vi "sub_filter_n_offset.vi"(8 "error in":errorcluster, 10 "offset?":bool, 11 "Q_data":T2) -> (0 "error out":errorcluster, 2 "data out":T1)   [LabVIEW 2013]
uses:
  ctl/q_data.ctl
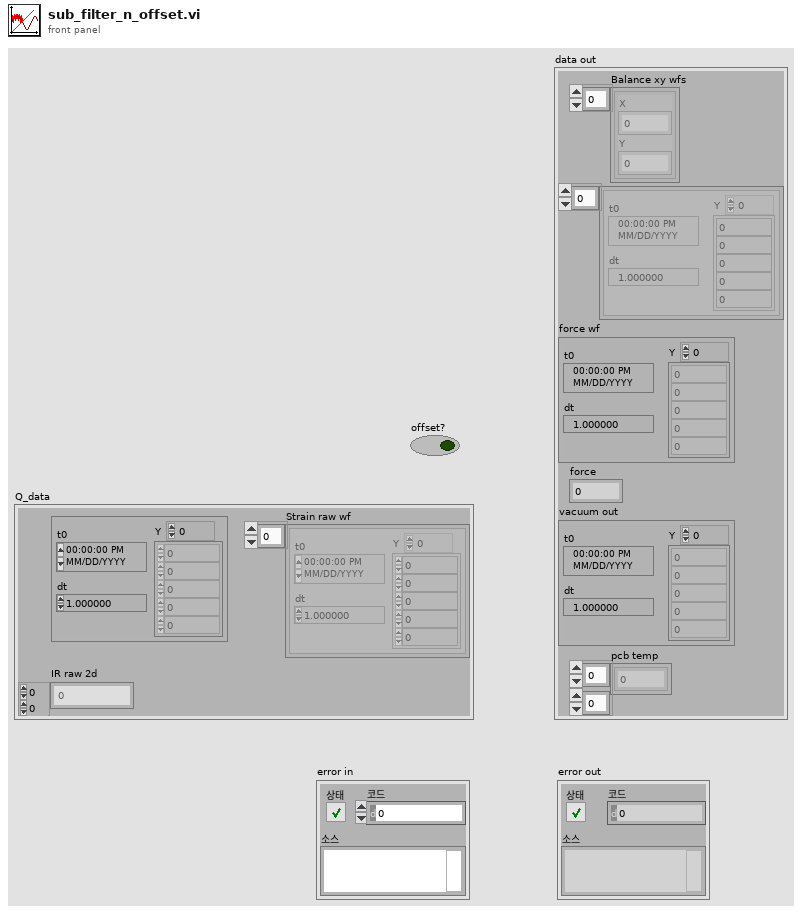
[diagram p1: front panel]
types:
  T1 = cluster{"Balance xy wfs":cluster{"X":dbl, "Y":dbl}[], waveform(dbl)[], "force wf":waveform(dbl), "force":dbl, "vacuum out":waveform(dbl), "pcb temp":dbl[][]}
  T2 = typedef "q_data.ctl" = cluster{"Strain raw wf":waveform(dbl)[], "vacuum raw wf":waveform(dbl), "IR raw 2d":i16[][]}
  T3 = typedef "config_ctl.ctl" = cluster{"Trigger minlevel":dbl, "Lower Cut-Off":dbl, "Vacuum Trigger level":dbl, "state settings":cluster{"method":enum32{"histogram", "peak", "auto select"}, "histogram size":i32, "histogram method":enum16{"mode"}, "reserved":dbl}, "SPA-300 Setting":cluster{"Bonding force (g)":dbl, "Bonding time (ms)":dbl, "Pickup force (g)":dbl, "Pickup time (ms)":dbl, "Speed":enum16{"Slow", "Fast"}}}
  T4 = typedef "UI_ctl.ctl" = cluster{"Heater temp":refnum<vi>, "heater":refnum<vi>, "vacuum (kpa)":refnum<vi>, "Balance xy graph":refnum<vi>, "Strain chart w cal":refnum<vi>, "Pickup force":refnum<vi>, "Pickup time":refnum<vi>, "Data chart":refnum<vi>, "Trigger graph":refnum<vi>, "vacuum 차트":refnum<vi>, "vacuum":refnum<vi>, "Strain raw graph":refnum<vi>, "Strain raw chart":refnum<vi>, "Bonding time":refnum<vi>, "Bonding force":refnum<vi>, "Balance":refnum<vi>, "Filtered force graph":refnum<vi>, "ROI intensity":refnum<vi>, "Heater_rt":refnum<vi>, "Tensile force":refnum<vi>, "Force rt":refnum<vi>}
  T5 = cluster{"Balance xy wfs":cluster{"X":dbl, "Y":dbl}[], waveform(dbl)[], "force wf":waveform(dbl), "force":dbl, "vacuum kpa wf":waveform(dbl), "pcb temp":dbl[][]}
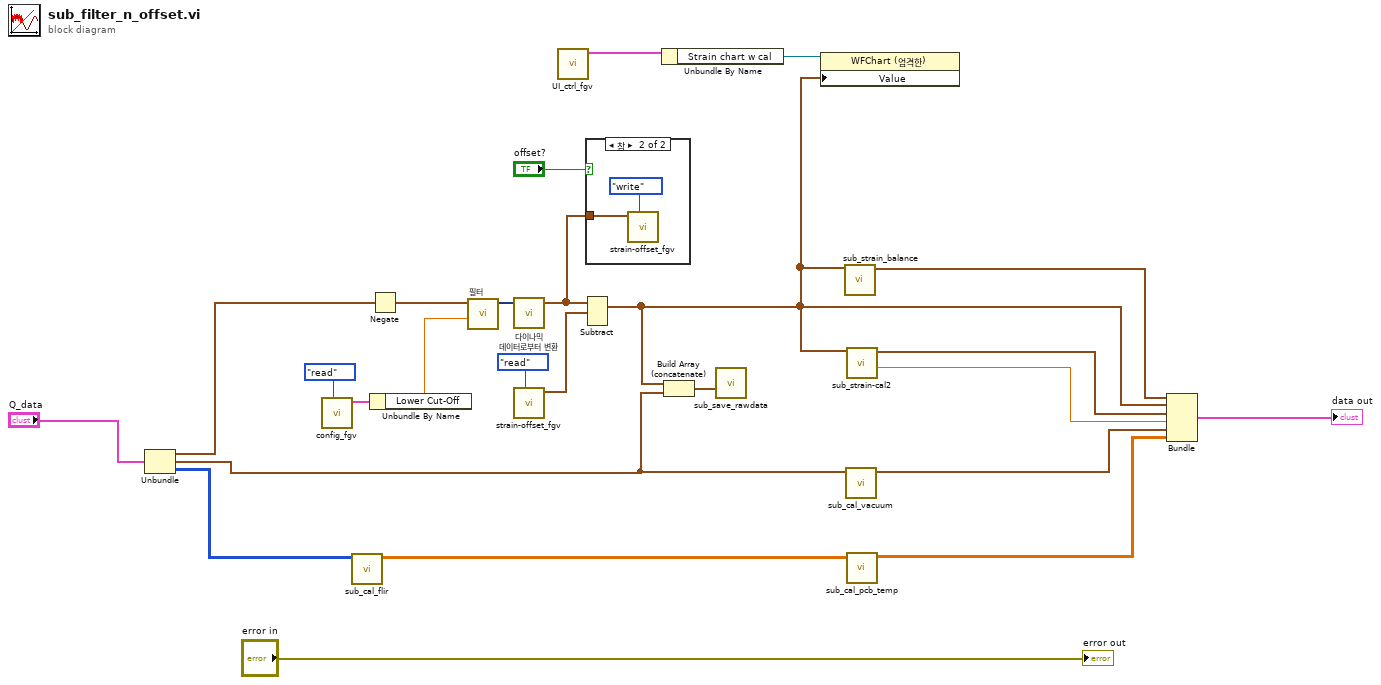
[diagram p0: block diagram]
diagram:
  n1 = Unbundle("Q_data") -> ("Strain raw wf"=w14:waveform(dbl)[], "vacuum raw wf"=w9:waveform(dbl), "IR raw 2d"=w13:i16[][])
  n2 = call "config_fgv.vi"("cmd"=enum16{"write", "read", "ini"}."read") -> ("Config out"=w18:T3)  [unwired: 9 in, 1 out]
  n3 = call "sub_cal_flir.vi"("FLIR cam data"=w13) -> ("temp data"=w12:dbl[][])  [unwired: 10 in]
  n4 = Negate(x=w14) -> (-x=w16:waveform(dbl)[])
  n5 = Unbundle By Name(w18) -> ("Lower Cut-Off"=w21:dbl)
  n6 = call "필터"("Lower Cut-Off"=w21, "Signal"=w16) -> ("Filtered Signal"=w20:dynamicdata)  [unwired: 8 in, 1 out]
  n7 = call "다이나믹 데이터로부터 변환"("Dynamic Data Type"=w20) -> ("Array of Waveform"=w23:waveform(dbl)[])  [unwired: 3 in]
  n8 = call "strain-offset_fgv.vi"("cmd"=enum16{"ini", "write", "read"}."read") -> ("Strain_offset_data"=w24:waveform(dbl)[])  [unwired: 10 in]
  n9 = call "UI_ctrl_fgv.vi"() -> ("UI cluster out"=w3:T4)  [unwired: 11 in]
  n10 = Subtract(1:w24, 2:w23) -> (0:w1:waveform(dbl)[])  [unwired: 1 in, 1 out]
  n11 = case shown="참" "offset?" {
    tunnel: w23 -> [_ w26]
    frame False {
    }
    frame True {
      n12 = call "strain-offset_fgv.vi"("cmd"=enum16{"ini", "write", "read"}."write", "data"=w26) -> ()  [unwired: 9 in, 1 out]
    }
  }
  n13 = Unbundle By Name(w3) -> ("Strain chart w cal"=w2:refnum<vi>)
  n14 = Build Array (concatenate)(w1, w9) -> (w17:waveform(dbl)[])
  n15 = call "sub_save_rawdata.vi"("배열"=w17) -> ()  [unwired: 10 in, 1 out]
  n16 = property class="WFChart (엄격한)"(reference=w2, "Value"=w1) -> ()  [unwired: 1 in, 2 out]
  n17 = call "sub_strain_balance.vi"("strain_offset_wf"=w1) -> ("Balance xy wfs"=w7:cluster{"X":dbl, "Y":dbl}[])  [unwired: 10 in]
  n18 = call "sub_cal_vacuum.vi"("vacuum v wf"=w9) -> ("vacuum kpa wf"=w8:waveform(dbl))  [unwired: 10 in]
  n19 = call "sub_strain-cal2.vi"("strain wfs"=w1) -> ("force"=w5:dbl, "force wf"=w6:waveform(dbl))  [unwired: 9 in]
  n20 = call "sub_cal_pcb_temp.vi"("ir temp"=w12) -> ("pcb temp"=w11:dbl[][])  [unwired: 10 in]
  n21 = Bundle("Balance xy wfs"=w7, w1, "force wf"=w6, "force"=w5, "vacuum kpa wf"=w8, "pcb temp"=w11) -> (→"data out":T5)  [unwired: 1 in]
  "error out" <- "error in"
